vi "Close Notifiers.vi"(8 "error in":errorcluster, 11 "Notifiers":T1) -> (0 "error out":errorcluster)   [LabVIEW 2015, in "Notifiers.lvlib"]
doc: "Releases notifiers"
uses:
  Notifiers.lvlib
  Notifiers.ctl
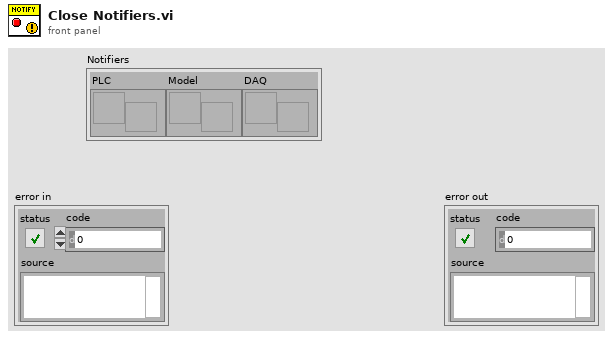
[diagram p1: front panel]
types:
  T1 = typedef "Notifiers.lvlib/Notifiers.ctl" = cluster{"PLC":refnum<notifier>, "Model":refnum<notifier>, "DAQ":refnum<notifier>}
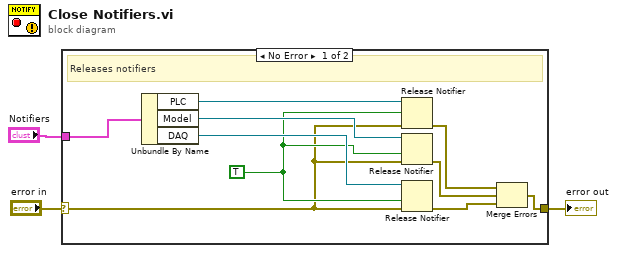
[diagram p0: block diagram]
diagram:
  n1 = case shown="No Error" "error in" {
    selector: "error in" -> [w4 w14]
    tunnel: [w10 w14] -> w2
    tunnel: "Notifiers" -> [w13 _]
    frame No Error {
      w5 = TRUE ("force destroy? (F)")
      # "Releases notifiers"
      n2 = Unbundle By Name(w13) -> ("PLC"=w12:refnum<notifier>, "Model"=w9:refnum<notifier>, "DAQ"=w7:refnum<notifier>)
      n3 = Release Notifier(notifier=w12, force destroy? (F)=w5, error in (no error)=w4) -> (error out=w11:errorcluster)  [unwired: 2 out]
      n4 = Release Notifier(notifier=w9, force destroy? (F)=w5, error in (no error)=w4) -> (error out=w8:errorcluster)  [unwired: 2 out]
      n5 = Release Notifier(notifier=w7, force destroy? (F)=w5, error in (no error)=w4) -> (error out=w6:errorcluster)  [unwired: 2 out]
      n6 = Merge Errors(w11, w8, w6) -> (w10:errorcluster)
    }
    frame Error {
    }
  }
  "error out" <- w2
